vi "Histeresis.vi"() -> ()   [LabVIEW 2015]
uses:
  <vilib>/Utility/file.llb/Read Delimited Spreadsheet (DBL).vi
panel:
  out "H percentage":dbl
  out "O increasing min":sgl
  out "O increasing max":sgl
  out "Hmax":dbl
  out "H":sgl[](array[numeric])
  out "out decreasing":sgl[](array[numeric])
  out "out increasing":sgl[](array[numeric])
  out "in (kg)":sgl[](array[numeric])
  in  "giriş sayısını giriniz":i32
  in  "ölçüm dosyası txt uzantılı":path
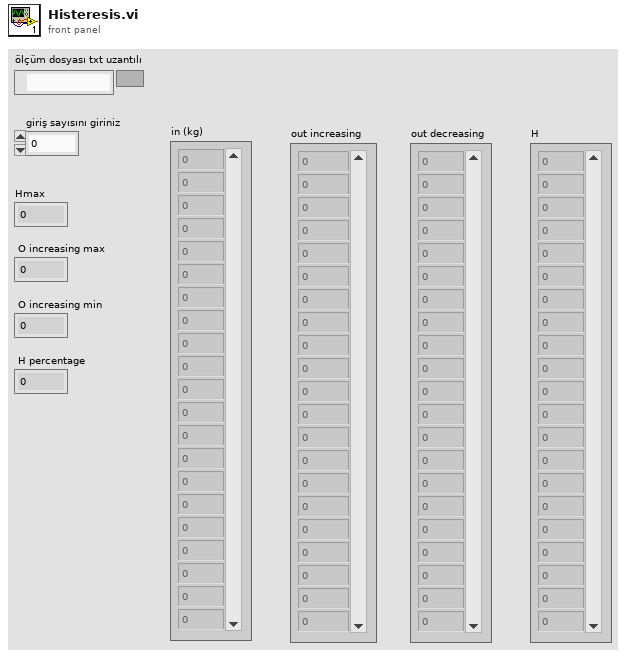
[diagram p1: front panel]
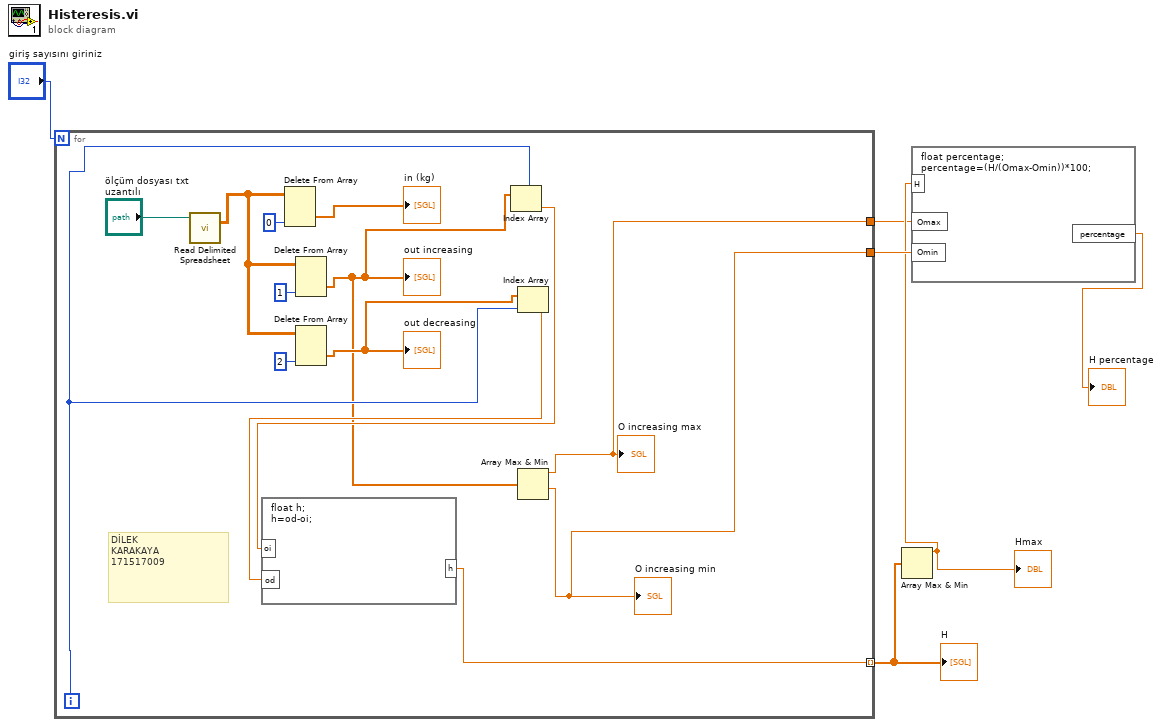
[diagram p0: block diagram]
diagram:
  n1 = for {
    N: "giriş sayısını giriniz" -> [_]
    tunnel: [w12] -> w4
    tunnel: [w11] -> w3 mode=indexing
    tunnel: [w10] -> w1
    i -> [w16]
    # "DİLEK \nKARAKAYA \n171517009"
    n2 = call-poly <vilib>:"Read Delimited Spreadsheet.vi"("file path (dialog if empty)"="ölçüm dosyası txt uzantılı") -> ("all rows"=w19:dbl[][])  [unwired: 9 in, 5 out]
    n3 = Delete From Array(array=w19, index (col)=0 ("disabled index (col)")) -> (deleted portion=→"in (kg)":dbl[])  [unwired: 2 in, 1 out]
    n4 = Delete From Array(array=w19, index (col)=1 ("disabled index (col)")) -> (deleted portion=w13:dbl[])  [unwired: 2 in, 1 out]
    "out increasing" <- w13
    n5 = Delete From Array(array=w19, index (col)=2 ("disabled index (col)")) -> (deleted portion=w17:dbl[])  [unwired: 2 in, 1 out]
    "out decreasing" <- w17
    n6 = Index Array(array=w13, index=w16) -> (element=w15:dbl)
    n7 = Index Array(array=w17, index=w16) -> (element=w14:dbl)
    n8 = formula code="float h;\nh=od-oi;"("oi"=w15, "od"=w14) -> ("h"=w11:dbl)
    n9 = Array Max & Min(array=w13) -> (max value=w10:dbl, min value=w12:dbl)  [unwired: 2 out]
    "O increasing max" <- w10
    "O increasing min" <- w12
  }
  "H" <- w3
  n10 = Array Max & Min(array=w3) -> (max value=w2:dbl)  [unwired: 3 out]
  "Hmax" <- w2
  n11 = formula code="float percentage;\npercentage=(H/(Omax-Omin))*100;"("H"=w2, "Omax"=w1, "Omin"=w4) -> ("percentage"=→"H percentage":dbl)
